vi "dashboard.vi"(8 "error in (no error)":errorcluster) -> (0 "error out":errorcluster)   [LabVIEW 2015]
uses:
  <vilib>/Rock Robotics/Network Tables/NT Write String Array.vi
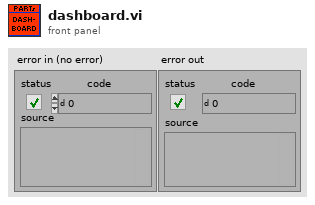
[diagram p1: front panel]
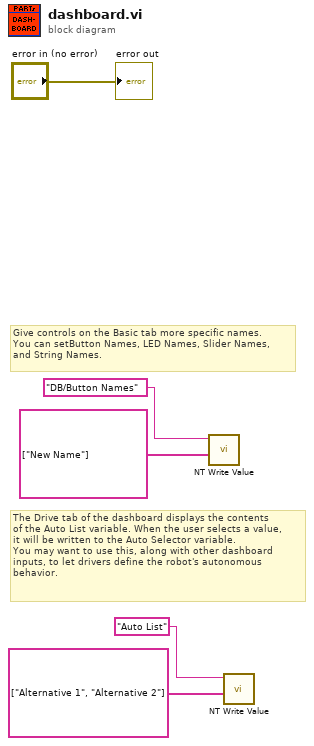
[diagram p0: block diagram]
diagram:
  # "The Drive tab of the dashboard displays the contents \nof the Auto List variable. When the user selects a value, \nit will be written to the Auto Selector variable. \nYou may want to use this, along with other dashboard \ninputs, to let drivers define the robot's autonomous\nbehavior."
  # "Give controls on the Basic tab more specific names. \nYou can setButton Names, LED Names, Slider Names,\nand String Names."
  n1 = call-poly <vilib>:"NT Write Value.vi"("String Array"=string[] ["New Name"], "Name"="DB/Button Names") -> ()  [unwired: 9 in, 1 out]
  n2 = call-poly <vilib>:"NT Write Value.vi"("String Array"=string[] ["Alternative 1", "Alternative 2"], "Name"="Auto List") -> ()  [unwired: 9 in, 1 out]
  "error out" <- "error in (no error)"
